vi "FPGA-Main.vi"() -> ()   [LabVIEW 2020]
doc: "This VI performs the I2C digital communication protocol on multiple user-defined ports."
uses:
  Controls/FPGA I2C_Cmd.ctl
  Controls/FPGA_I2C IO Cluster.ctl
  Controls/FPGA I2C_Comm Loop State.ctl
  <vilib>/rvi/Emulation/niFpgaGetClockAttributes.vi
  <vilib>/rvi/Emulation/niFpgaSctlEmulationGetInTimedLoop.vi
  <vilib>/rvi/Emulation/niFpgaEmulationReportErrorSimple.vi
  <vilib>/rvi/Emulation/niFpgaCriticalErrorInLSC.vi
  FPGA SubVIs/FPGA_I2C_Globals.vi
  <vilib>/rvi/Emulation/niFpgaProcessEmulError.vi
  <vilib>/rvi/Emulation/niFpgaEmulationIsFPGAContextNoSignature.vi
  <vilib>/rvi/errors/niFpgaSetErrorForExecOnDevCompSimple.vi
  <vilib>/rvi/eio/common/nirviEmuReportErrorAndStop.vi
  <vilib>/rvi/DataTransferAndStorage/Container/Common/niFpgaContainerGetUniqueNameForEmu.vi
  <vilib>/rvi/FIFO/Fifo_Resource/nirvififoEmulationSetSize.vi
  <vilib>/rvi/FIFO/Fifo_Resource/nirviFifoEmulationQueueMgr.vi
  <instcachedir>/0/nirviFifoEmulationQueueMgr_E5CAEC123FF24DC58D834DCA3CDAA9B5.lvgen/nirviFifoEmulationQueueMgr_E5CAEC123FF24DC58D834DCA3CDAA9B5_001.vi
  <vilib>/rvi/FIFO/Fifo_Resource/nirvififoEmulationDetermineInputValidOut.vi
  <vilib>/rvi/FIFO/Fifo_Resource/nirvififoEmulationCreateLock.vi
  <vilib>/rvi/FIFO/Fifo_Resource/nirvififoEmulationObtainLock.vi
  <vilib>/rvi/FIFO/Fifo_Resource/nirvififoEmulationReleaseLock.vi
  <vilib>/rvi/occurrence/nirviWaitOnOccurrenceBase.vi
  <vilib>/rvi/errors/nirviReportUnexpectedCaseInternalError.vi
  <vilib>/rvi/errors/nirviReportUnexpectedCaseInternalError (U32).vi
  <vilib>/Utility/error.llb/Clear Errors.vi
  <vilib>/rvi/DataTransferAndStorage/Container/XNode/niFpgaContainer.xnode
  <vilib>/rvi/FIFO/Fifo_Resource/nirvififoEmulationWrite.vi
  <vilib>/rvi/FIFO/Fifo_Resource/nirvififoEmulationRead.vi
panel:
  out "Error Out":errorcluster
  out "ROM Data":u8[](array[numeric]) format="%.0x"
  in  "Error In":errorcluster
  out "Scratchpad Data":u8[](array[numeric]) format="%.0x"
  out "Loop Rate (tics)":u32
  in  "I2C_Address":u16
  in  "I2C_Bytes to Read":u16=1
  in  "I2C_Bytes to Write":u16=1
  in  "I2C_Wait Time/2":u32=200
  in  "I2C_Wait Time":u32=400
  in  "I2C_Port":u8
  in  "I2C_Ack Read":bool
  out "I2C_Read Flag":bool
  out "I2C_Read Data":u8
  in  "I2C_Write Data":u8
  in  "I2C_Write Flag":bool
  in  "I2C_Cmd":T1
  in  "I2C_Start":bool
  # "Pressure Sensor"
  # "Control"
  # "I2C Parameters"
  # "Command Type"
  # "Host Data Transfer"
  # "Temperature Sensor"
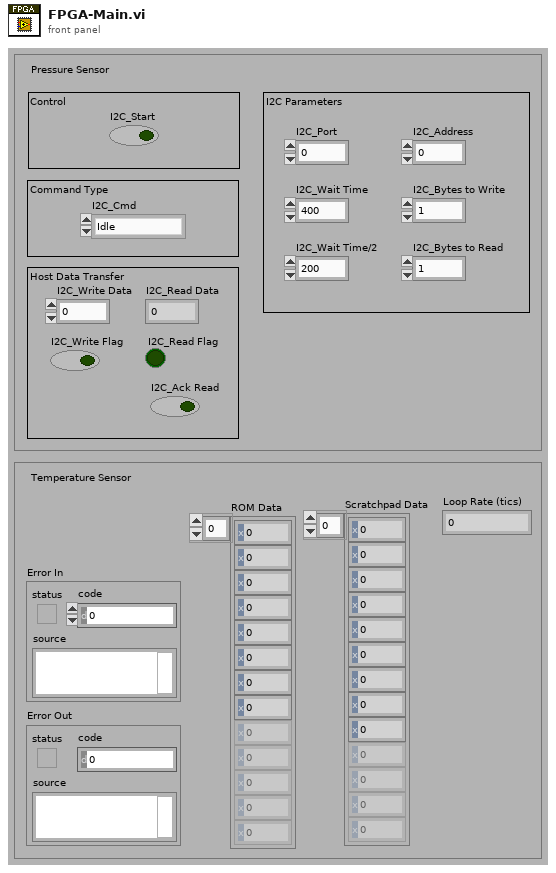
[diagram p1: front panel]
types:
  T1 = typedef "FPGA I2C_Cmd.ctl" = enum8{"Idle", "Write I2C", "Read I2C", "Write & Read I2C", "Configure"}
  T2 = typedef "FPGA I2C_Comm Loop State.ctl" = enum8{"Idle", "Init", "Write", "Start", "Read", "Wait Until Done"}
  T3 = typedef "FPGA_I2C IO Cluster.ctl" = cluster{"SCK":refnum<k21>, "DATA":refnum<k21>}
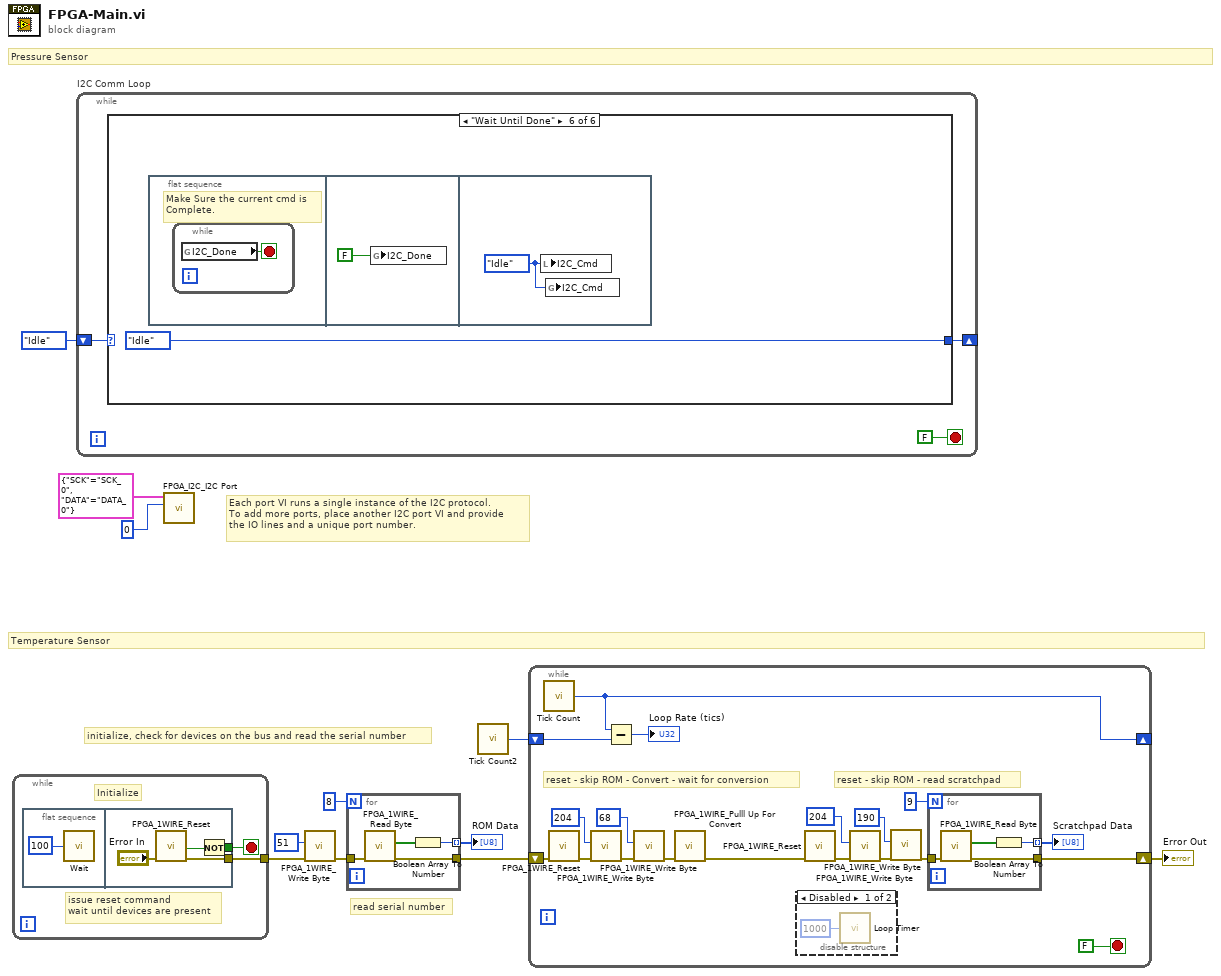
[diagram p0: block diagram]
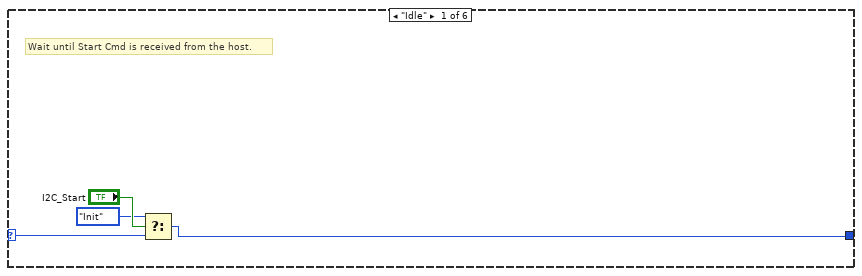
[diagram p3: hidden frame]
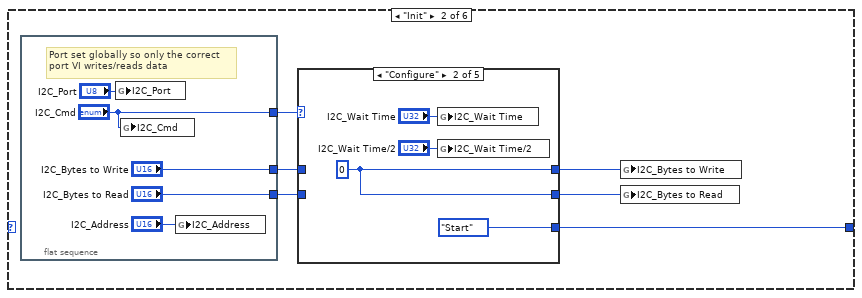
[diagram p4: hidden frame]
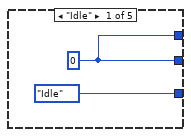
[diagram p5: hidden frame]
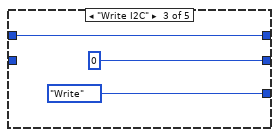
[diagram p6: hidden frame]
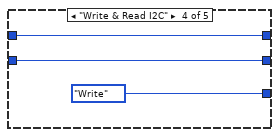
[diagram p7: hidden frame]
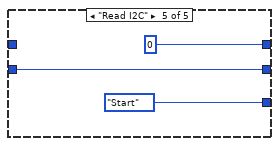
[diagram p8: hidden frame]
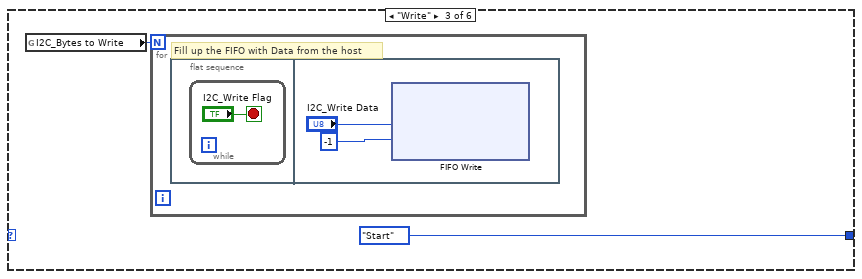
[diagram p9: hidden frame]
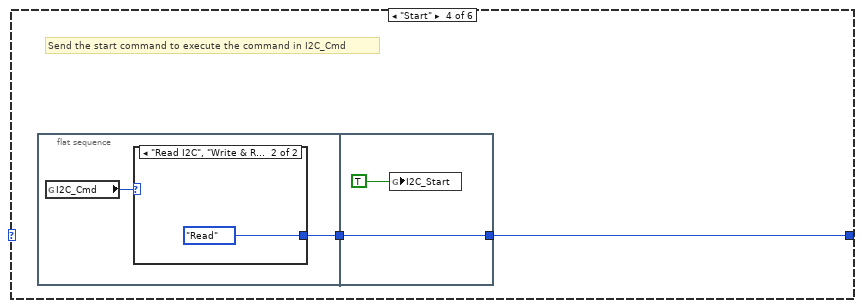
[diagram p10: hidden frame]
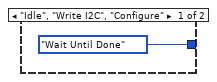
[diagram p11: hidden frame]
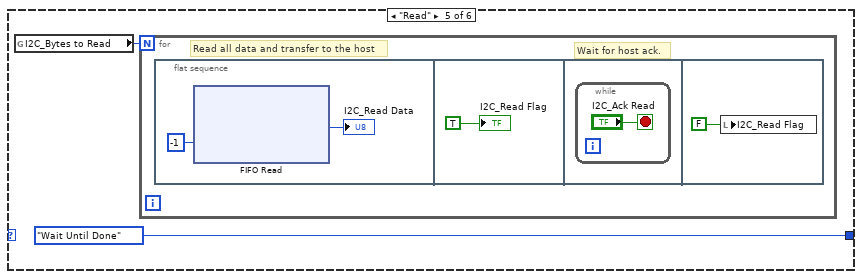
[diagram p12: hidden frame]
diagram:
  # "read serial number"
  # "initialize, check for devices on the bus and read the serial number"
  # "Temperature Sensor"
  # "Pressure Sensor"
  # "Each port VI runs a single instance of the I2C protocol.\nTo add more ports, place another I2C port VI and provide\nthe IO lines and a unique port number."
  n1 = while {
    tunnel: [w12] -> w3
    stop <- w13 stop-if-true
    # "Initialize"
    # "issue reset command\nwait until devices are present"
    n2 = flat-sequence {
      tunnel: [w18] -> w13
      tunnel: [w16] -> w12
      frame #0 {
        n3 = call "Wait"("Count(mSec)"=u32 100) -> ()  [unwired: 1 out]
      }
      frame #1 {
        n4 = call "FPGA_1WIRE_Reset.vi"("error in"="Error In") -> ("error out"=w16:errorcluster, "0 = Device Present / 1=no"=w15:bool)  [unwired: 9 in]
        n5 = Not(x=w15) -> (.not. x?=w18:bool)
      }
    }
  }
  n6 = while "I2C Comm Loop" {
    shift-right: [w20] -> _
    shift-left: FPGA_I2C_Comm_Loop_State."Idle" ("Action") -> [w19]
    stop <- FALSE stop-if-true
    n7 = case shown="\"Wait Until Done\"" w19 {
      selector: w19 -> [w24 _ _ _ _ _]
      tunnel: [w22 w30 FPGA_I2C_Comm_Loop_State."Start" ("Action") w58 FPGA_I2C_Comm_Loop_State."Wait Until Done" ("Action") FPGA_I2C_Comm_Loop_State."Idle" ("Action")] -> w20
      frame "Idle" {
        # "Wait until Start Cmd is received from the host."
        n8 = Select(t=FPGA_I2C_Comm_Loop_State."Init" ("Action"), s="I2C_Start", f=w24) -> (s? t:f=w22:T2)
      }
      frame "Init" {
        n9 = flat-sequence {
          tunnel: ["I2C_Cmd"] -> w31
          tunnel: ["I2C_Bytes to Write"] -> w29
          tunnel: ["I2C_Bytes to Read"] -> w27
          frame #0 {
            # "Port set globally so only the correct\nport VI writes/reads data"
            n10 = global write "FPGA_I2C_Globals.vi" "I2C_Port"("I2C_Port") -> ()
            n11 = global write "FPGA_I2C_Globals.vi" "I2C_Cmd"("I2C_Cmd") -> ()
            n12 = global write "FPGA_I2C_Globals.vi" "I2C_Address"("I2C_Address") -> ()
          }
        }
        n13 = case shown="\"Configure\"" w31 {
          tunnel: [FPGA_I2C_Comm_Loop_State."Idle" ("Action") FPGA_I2C_Comm_Loop_State."Start" ("Action") FPGA_I2C_Comm_Loop_State."Write" ("Action") FPGA_I2C_Comm_Loop_State."Write" ("Action") FPGA_I2C_Comm_Loop_State."Start" ("Action")] -> w30
          tunnel: [w37 w39 w44 w47 u16 0 ("I2C_Bytes to Read")] -> w28
          tunnel: w29 -> [_ _ w44 w47 _]
          tunnel: w27 -> [_ _ _ w46 w49]
          tunnel: [w37 w39 u16 0 ("I2C_Bytes to Read") w46 w49] -> w26
          frame "Idle" {
            w37 = u16 0 ("I2C_Bytes to Read")
          }
          frame "Configure" {
            w39 = u16 0 ("I2C_Bytes to Read")
            n14 = global write "FPGA_I2C_Globals.vi" "I2C_Wait Time"("I2C_Wait Time") -> ()
            n15 = global write "FPGA_I2C_Globals.vi" "I2C_Wait Time/2"("I2C_Wait Time/2") -> ()
          }
          frame "Write I2C" {
          }
          frame "Write & Read I2C" {
          }
          frame "Read I2C" {
          }
        }
        n16 = global write "FPGA_I2C_Globals.vi" "I2C_Bytes to Write"(w28) -> ()
        n17 = global write "FPGA_I2C_Globals.vi" "I2C_Bytes to Read"(w26) -> ()
      }
      frame "Write" {
        n18 = global read "FPGA_I2C_Globals.vi" "I2C_Bytes to Write"() -> (w52:u16)
        n19 = for {
          N: w52 -> [_]
          # "Fill up the FIFO with Data from the host"
          n20 = flat-sequence {
            frame #0 {
              n21 = while {
                stop <- "I2C_Write Flag" stop-if-true
              }
            }
            frame #1 {
              n22 = xnode ("FIFO Write")("Element"="I2C_Write Data", "Timeout"=-1) -> ()  [unwired: 1 in, 2 out]
            }
          }
        }
      }
      frame "Start" {
        # "Send the start command to execute the command in I2C_Cmd"
        n23 = flat-sequence {
          tunnel: [w60] -> w57
          tunnel: [w64] -> w58
          tunnel: w57 -> [w64]
          frame #0 {
            n24 = global read "FPGA_I2C_Globals.vi" "I2C_Cmd"() -> (w59:T1)
            n25 = case shown="\"Read I2C\", \"Write & Read I2C\"" w59 {
              tunnel: [FPGA_I2C_Comm_Loop_State."Wait Until Done" ("Action") FPGA_I2C_Comm_Loop_State."Read" ("Action")] -> w60
              frame "Idle", "Write I2C", "Configure" {
              }
              frame "Read I2C", "Write & Read I2C" {
              }
            }
          }
          frame #1 {
            n26 = global write "FPGA_I2C_Globals.vi" "I2C_Start"(TRUE ("Write Flag")) -> ()
          }
        }
      }
      frame "Read" {
        n27 = global read "FPGA_I2C_Globals.vi" "I2C_Bytes to Read"() -> (w65:u16)
        n28 = for {
          N: w65 -> [_]
          # "Wait for host ack."
          # "Read all data and transfer to the host"
          n29 = flat-sequence {
            frame #0 {
              n30 = xnode ("FIFO Read")("Timeout"=-1) -> ("Element"=→"I2C_Read Data":u8)  [unwired: 1 in, 2 out]
            }
            frame #1 {
              "I2C_Read Flag" <- TRUE ("Read Flag")
            }
            frame #2 {
              n31 = while {
                stop <- "I2C_Ack Read" stop-if-true
              }
            }
            frame #3 {
              n32 = local write "I2C_Read Flag"(FALSE ("Read Flag")) -> ()
            }
          }
        }
      }
      frame "Wait Until Done" {
        n33 = flat-sequence {
          frame #0 {
            # "Make Sure the current cmd is\nComplete."
            n34 = while {
              stop <- w73 stop-if-true
              n35 = global read "FPGA_I2C_Globals.vi" "I2C_Done"() -> (w73:bool)
            }
          }
          frame #1 {
            n36 = global write "FPGA_I2C_Globals.vi" "I2C_Done"(FALSE ("Done")) -> ()
          }
          frame #2 {
            w75 = FPGA_I2C_Cmd."Idle" ("I2C_Cmd")
            n37 = local write "I2C_Cmd"(w75) -> ()
            n38 = global write "FPGA_I2C_Globals.vi" "I2C_Cmd"(w75) -> ()
          }
        }
      }
    }
  }
  n39 = call "FPGA_I2C_I2C Port.vi"("Port"=u8 0, "IO Cluster"=T3 {"SCK"="SCK_0", "DATA"="DATA_0"}) -> ()  [unwired: 10 out]
  n40 = call "FPGA_1WIRE_Write Byte.vi"("error in"=w3, "Tx data"=u8 51 ("Tx data 2")) -> ("error out"=w1:errorcluster)  [unwired: 8 in, 1 out]
  n41 = for {
    N: 8 -> [_]
    tunnel: [w77] -> w4
    tunnel: [w79] -> w8 mode=indexing
    tunnel: w1 -> [w78]
    n42 = call "FPGA_1WIRE_Read Byte.vi"("error in"=w78) -> ("error out"=w77:errorcluster, "Array"=w76:bool[])  [unwired: 9 in]
    n43 = Boolean Array To Number(Boolean array=w76) -> (number=w79:u8)
  }
  "ROM Data" <- w8
  n44 = call "Tick Count2"() -> ("Tick Count(Ticks)"=w6:u32)
  n45 = while {
    shift-right: [w94] -> _
    shift-left: w6 -> [w95]
    shift-right: [w92] -> w5
    shift-left: w4 -> [w91]
    stop <- FALSE ("stop") stop-if-true
    # "reset - skip ROM - read scratchpad"
    # "reset - skip ROM - Convert - wait for conversion"
    n46 = call "Tick Count"() -> ("Tick Count(Ticks)"=w94:u32)
    n47 = call "FPGA_1WIRE_Reset.vi"("error in"=w91) -> ("error out"=w89:errorcluster)  [unwired: 9 in, 1 out]
    n48 = call "FPGA_1WIRE_Write Byte.vi"("error in"=w89, "Tx data"=u8 204) -> ("error out"=w86:errorcluster)  [unwired: 8 in, 1 out]
    n49 = Subtract(x=w94, y=w95) -> (x-y=→"Loop Rate (tics)":u32)
    n50 = call "FPGA_1WIRE_Write Byte.vi"("error in"=w86, "Tx data"=u8 68 ("Tx data 2")) -> ("error out"=w87:errorcluster)  [unwired: 8 in, 1 out]
    n51 = call "FPGA_1WIRE_Pulll Up For Convert.vi"("error in"=w87) -> ("error out"=w90:errorcluster)  [unwired: 10 in]
    n52 = disable-structure shown="Disabled" {
      frame Disabled {
        n53 = call "Loop Timer"("Count(mSec)"=u32 1000) -> ()  [unwired: 1 out]
      }
      frame Enabled {
      }
    }
    n54 = call "FPGA_1WIRE_Reset.vi"("error in"=w90) -> ("error out"=w84:errorcluster)  [unwired: 9 in, 1 out]
    n55 = call "FPGA_1WIRE_Write Byte.vi"("error in"=w84, "Tx data"=u8 204) -> ("error out"=w82:errorcluster)  [unwired: 8 in, 1 out]
    n56 = call "FPGA_1WIRE_Write Byte.vi"("error in"=w82, "Tx data"=u8 190 ("Tx data 2")) -> ("error out"=w80:errorcluster)  [unwired: 8 in, 1 out]
    n57 = for {
      N: 9 -> [_]
      tunnel: [w101] -> w92
      tunnel: [w103] -> w96 mode=indexing
      tunnel: w80 -> [w102]
      n58 = call "FPGA_1WIRE_Read Byte.vi"("error in"=w102) -> ("error out"=w101:errorcluster, "Array"=w100:bool[])  [unwired: 9 in]
      n59 = Boolean Array To Number(Boolean array=w100) -> (number=w103:u8)
    }
    "Scratchpad Data" <- w96
  }
  "Error Out" <- w5
